vi "Read Client ID.vi"(8 "error in (no error)":errorcluster, 11 "Client in":refnum<class "SC-Client.lvclass">) -> (0 "error out":errorcluster, 2 "Client ID":i32, 3 "Client out":refnum<class "SC-Client.lvclass">)   [LabVIEW 2013, in "SLMControl.lvlib" / "SC-Client.lvclass"]
uses:
  SC-Client.lvclass
  SC-Client.lvclass/SC-Client.ctl
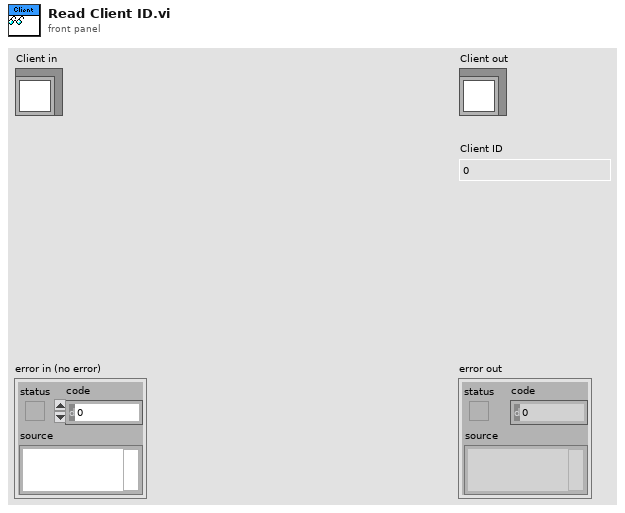
[diagram p1: front panel]
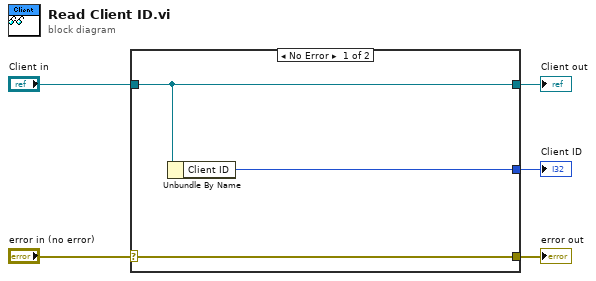
[diagram p0: block diagram]
diagram:
  n1 = case shown="No Error" "error in (no error)" {
    selector: "error in (no error)" -> [w8 w9]
    tunnel: [w8 w9] -> w4
    tunnel: [w7 w10] -> w2
    tunnel: "Client in" -> [w7 w10]
    tunnel: [w6 _] -> w1
    frame No Error {
      n2 = Unbundle By Name(w7) -> ("Client ID"=w6:i32)
    }
    frame Error {
    }
  }
  "error out" <- w4
  "Client out" <- w2
  "Client ID" <- w1
